vi "DisposeCore.vi"(8 "error in (no error)":errorcluster, 11 "ConcreteCreatorA in":refnum<class "ConcreteCreatorA.lvclass">) -> (0 "error out":errorcluster, 3 "ConcreteCreatorA out":refnum<class "ConcreteCreatorA.lvclass">)   [LabVIEW 2020, in "FactoryMethod.lvlib" / "ConcreteCreatorA.lvclass"]
uses:
  ConcreteCreatorA.lvclass
  Private/TypeDef/privateDataDVR.ctl
  Private/TypeDef/privateData.ctl
  ConcreteCreatorA.lvclass/ConcreteCreatorA.ctl
  Creator/Creator.lvclass
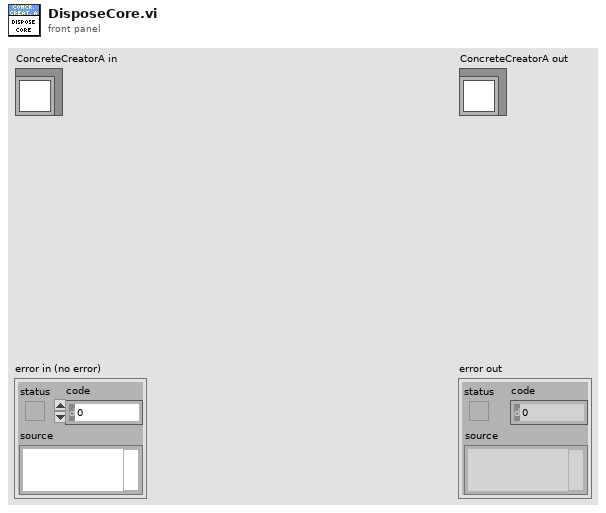
[diagram p1: front panel]
types:
  T1 = typedef "FactoryMethod.lvlib/ConcreteCreatorA.lvclass/privateDataDVR.ctl" = refnum<data-value>
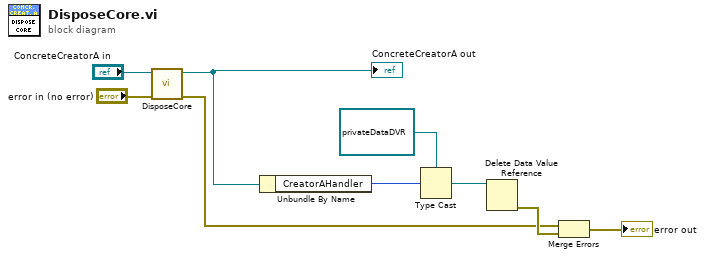
[diagram p0: block diagram]
diagram:
  n1 = call-parent "DisposeCore.vi"("error in (no error)"="error in (no error)", "Creator in"="ConcreteCreatorA in") -> ("error out"=w2:errorcluster, "Creator out"=w1:refnum<class "ConcreteCreatorA.lvclass">)  [unwired: 8 in]
  "ConcreteCreatorA out" <- w1
  n2 = Unbundle By Name(w1) -> ("CreatorAHandler"=w6:u32)
  n3 = Type Cast(type=T1 refnum ("privateDataDVR"), x=w6) -> (*(type *) &x=w7:T1)
  n4 = Delete Data Value Reference(data value reference=w7) -> (error out=w4:errorcluster)  [unwired: 1 in, 1 out]
  n5 = Merge Errors(w2, w4) -> (→"error out":errorcluster)
